vi "Main.vi"   [LabVIEW 2020, in "LV-Term App.lvclass"]
uses:
  LV-Term App.lvclass
  LV-Term App.lvclass/LV-Term App.ctl
panel:
  # "LV-Term\nApp\nMain"
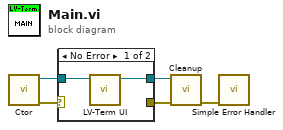
[diagram p0: block diagram]
diagram:
  n1 = call "Ctor.vi"() -> ("error out"=w4:errorcluster, "LV-Term App out"=w5:refnum<class "LV-Term App.lvclass">)  [unwired: 10 in]
  n2 = case shown="No Error" w4 {
    selector: w4 -> [_ w9]
    tunnel: w5 -> [w7 w8]
    tunnel: [w6 w8] -> w3
    tunnel: [_ w9] -> w2
    frame No Error {
      n3 = call "LV-Term UI.vi"("LV-Term App In"=w7) -> ("LV-Term App"=w6:refnum<class "LV-Term App.lvclass">)  [unwired: 10 in]
    }
    frame Error {
    }
  }
  n4 = call "Cleanup.vi"("error in (no error)"=w2, "LV-Term App in"=w3) -> ("error out"=w1:errorcluster)  [unwired: 9 in]
  n5 = call <vilib>:"Simple Error Handler.vi"("error in (no error)"=w1) -> ()  [unwired: 4 in, 5 out]
